vi "Resolve Headers.vi"(8 "error in (no error)":errorcluster, 10 "headers in":T1[](array[typedef]), 11 "REST Client in":refnum<class "REST Client.lvclass">) -> (0 "error out":errorcluster, 2 "headers out":T1[](array[typedef]), 3 "REST Client out":refnum<class "REST Client.lvclass">)   [LabVIEW 2018, in "REST Client_JKI.lvlib" / "REST Client.lvclass"]
uses:
  REST Client.lvclass
  HTTP Header.ctl
  REST Client.lvclass/REST Client.ctl
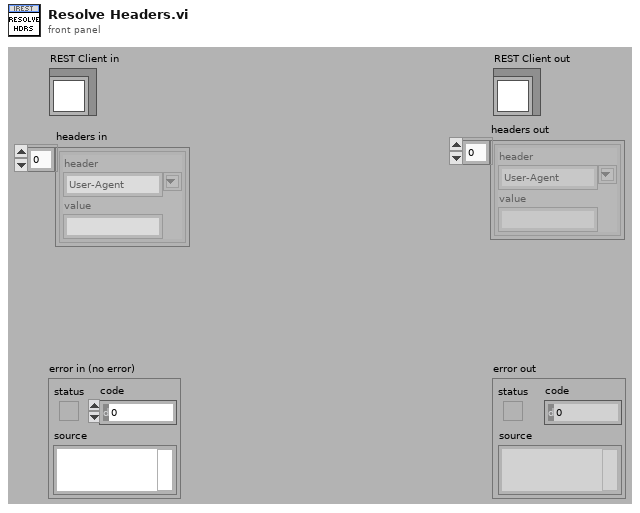
[diagram p1: front panel]
types:
  T1 = typedef "REST Client_JKI.lvlib/REST Client.lvclass/HTTP Header.ctl" = cluster{"header":string, "value":string}
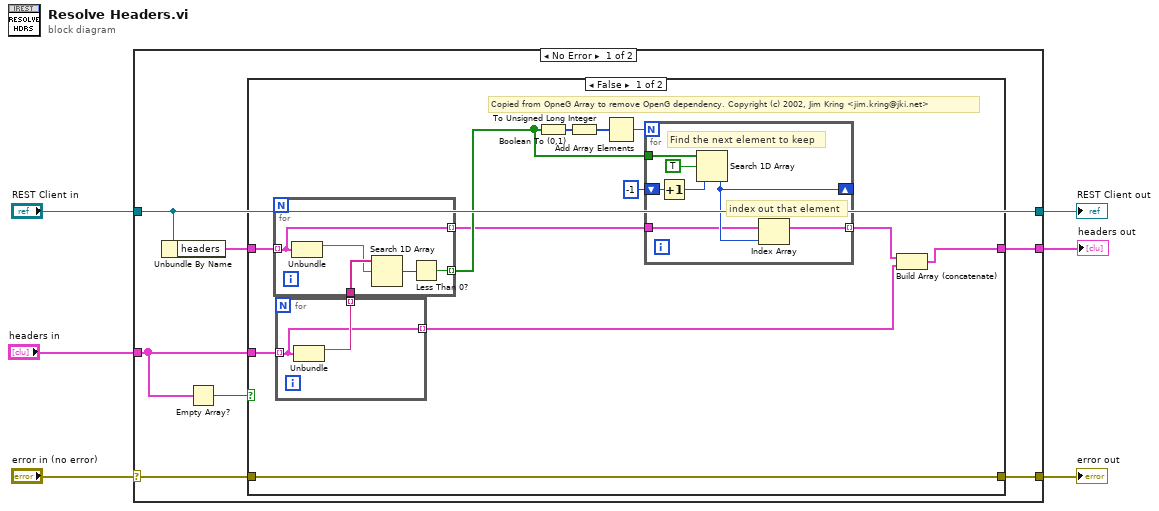
[diagram p0: block diagram]
diagram:
  n1 = case shown="No Error" "error in (no error)" {
    selector: "error in (no error)" -> [w8 w44]
    tunnel: [w7 w44] -> w5
    tunnel: [w13 w43] -> w3
    tunnel: "REST Client in" -> [w13 w43]
    tunnel: "headers in" -> [w11 _]
    tunnel: [w9 _] -> w1
    frame No Error {
      n2 = Unbundle By Name(w13) -> ("headers"=w10:cluster{"header":string, "value":string}[])
      n3 = Empty Array?(array=w11) -> (empty?=w12:bool)
      n4 = case shown="False" w12 {
        tunnel: w11 -> [w25 _]
        tunnel: w10 -> [w26 w42]
        tunnel: [w23 w42] -> w9
        tunnel: w8 -> [w14 w41]
        tunnel: [w14 w41] -> w7
        frame False {
          # "Copied from OpneG Array to remove OpenG dependency. Copyright (c) 2002, Jim Kring <jim.kring@jki.net>"
          n5 = for {
            tunnel: w25 -> [w34] mode=indexing
            tunnel: [w35] -> w24 mode=indexing
            tunnel: [w34] -> w22 mode=indexing
            n6 = Unbundle(w34) -> ("header"=w35:string)  [unwired: 1 out]
          }
          n7 = for {
            tunnel: w26 -> [w36] mode=indexing
            tunnel: w24 -> [w40]
            tunnel: [w37] -> w17 mode=indexing
            tunnel: [w36] -> w16 mode=indexing
            n8 = Unbundle(w36) -> ("header"=w39:string)  [unwired: 1 out]
            n9 = Search 1D Array(1D array=w40, element=w39) -> (index of element=w38:i32)  [unwired: 1 in]
            n10 = Less Than 0?(x=w38) -> (x < 0?=w37:bool)
          }
          n11 = Boolean To (0,1)(Boolean=w17) -> (0, 1=w19:i16[])
          n12 = To Unsigned Long Integer(number=w19) -> (unsigned 32bit integer=w18:u32[])
          n13 = Add Array Elements(numeric array=w18) -> (sum=w20:u32)
          n14 = for {
            N: w20 -> [_]
            tunnel: w16 -> [w29]
            tunnel: w17 -> [w33]
            shift-right: [w30] -> _
            shift-left: -1 ("start index (0)") -> [w31]
            tunnel: [w28] -> w15 mode=indexing
            # "index out that element"
            # "Find the next element to keep"
            n15 = Increment(x=w31) -> (x+1=w27:i32)
            n16 = Search 1D Array(1D array=w33, element=TRUE, start index (0)=w27) -> (index of element=w30:i32)
            n17 = Index Array(array=w29, index=w30) -> (element=w28:cluster{"header":string, "value":string})
          }
          n18 = Build Array (concatenate)(w15, w22) -> (w23:T1[])
        }
        frame True {
        }
      }
    }
    frame Error {
    }
  }
  "error out" <- w5
  "REST Client out" <- w3
  "headers out" <- w1
